vi "Get FPGA Reference.vi"(8 "error in (no error)":errorcluster, 11 "nCRD in":refnum<class "gCRD.lvclass">) -> (0 "error out":errorcluster, 2 "FPGA Ref":T1, 3 "nCRD out":refnum<class "gCRD.lvclass">)   [LabVIEW 2016, in "gCRDS.lvlib" / "gCRD.lvclass"]
uses:
  gCRD.lvclass
  Session/Raw FPGA/FPGA Session.lvclass
  FPGA Ref.ctl
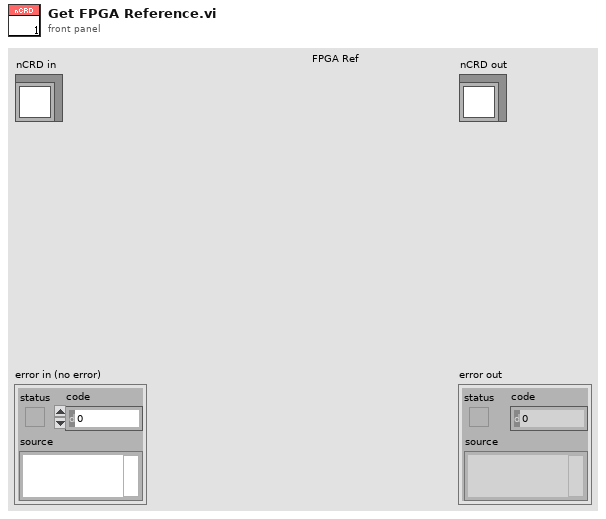
[diagram p1: front panel]
types:
  T1 = typedef "FPGA Ref.ctl" = refnum<k20>
  T2 = typedef "Session - Root.lvclass/Session Handle.ctl" = refnum<data-value>
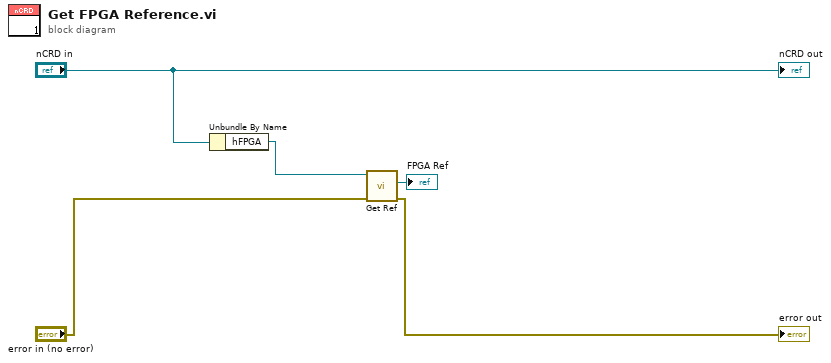
[diagram p0: block diagram]
diagram:
  n1 = Unbundle By Name("nCRD in") -> ("hFPGA"=w4:T2)
  n2 = call "Get Ref.vi"("error in"="error in (no error)", "Hanlde Out"=w4) -> ("error out"=→"error out":errorcluster, "FPGA Ref"=→"FPGA Ref":T1)  [unwired: 7 in, 1 out]
  "nCRD out" <- "nCRD in"
